vi "Shift Fwd.vi"(11 "Circular Buffer in":refnum<class "Circular Buffer.lvclass">) -> (3 "Circular Buffer out":refnum<class "Circular Buffer.lvclass">)   [LabVIEW 2023, in "d20.lvlib" / "Circular Buffer.lvclass"]
uses:
  Circular Buffer.lvclass
  Circular Buffer.lvclass/Circular Buffer.ctl
  INode/INode.lvclass
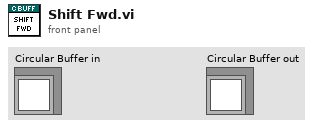
[diagram p1: front panel]
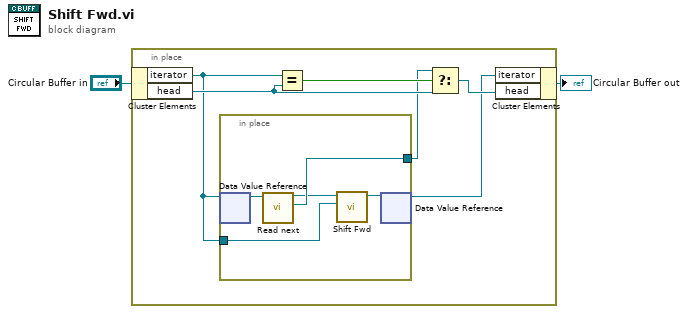
[diagram p0: block diagram]
diagram:
  n1 = in-place {
    n2 = in-place-cluster #1("Circular Buffer in") -> ("iterator"=w3:refnum<data-value>, "head"=w7:refnum<data-value>)
    n3 = in-place {
      in-place-border: w3 -> [w11]
      in-place-border: [w13] -> w4
      n4 = in-place-dvr #2(w3) -> (w9:refnum<class "INode.lvclass">)  [unwired: 1 out]
      n5 = call-dynamic "Read next.vi"("Node in"=w9) -> ("next"=w13:refnum<data-value>, "Node out"=w12:refnum<class "INode.lvclass">)  [unwired: 9 in]
      n6 = call-dynamic "Shift Fwd.vi"("iterator"=w11, "INode in"=w12) -> ("INode out"=w10:refnum<class "INode.lvclass">)  [unwired: 9 in]
      n7 = in-place-dvr #2(w10) -> (w5:refnum<data-value>)  [unwired: 1 out]
    }
    n8 = Equal?(x=w3, y=w7) -> (x = y?=w8:bool)
    n9 = Select(t=w4, s=w8, f=w7) -> (s? t:f=w6:refnum<data-value>)
    n10 = in-place-cluster #1("iterator"=w5, "head"=w6) -> (→"Circular Buffer out":refnum<class "Circular Buffer.lvclass">)
  }
